vi "get_screen_resolution.vi"() -> (0 "Vertical Offset":i32, 1 "Height pixels":i16, 2 "Width pixels":i16)   [LabVIEW 2018]
uses:
  user32.dll
panel:
  out "Taskbar Height":i16
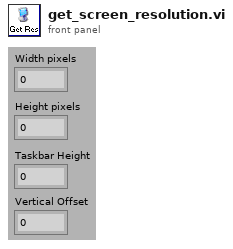
[diagram p1: front panel]
types:
  T1 = typedef "LVAllMonitorsDisplayTypeDef.ctl" = cluster{"Bounds":cluster{"Left":i16, "Top":i16, "Right":i16, "Bottom":i16}, "Depth":i16}[]
  T2 = typedef "LVRectTypeDef.ctl" = cluster{"Left":i16, "Top":i16, "Right":i16, "Bottom":i16}
  T3 = cluster{"Bounds":cluster{"Left":i16, "Top":i16, "Right":i16, "Bottom":i16}, "Depth":i16}
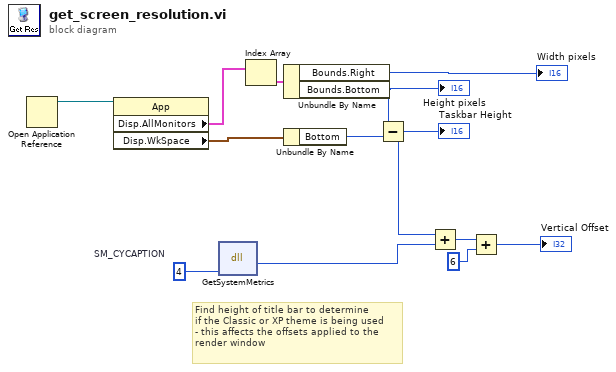
[diagram p0: block diagram]
diagram:
  w8 = 4  # SM_CYCAPTION
  # "Find height of title bar to determine\nif the Classic or XP theme is being used\n- this affects the offsets applied to the\nrender window"
  n1 = Open Application Reference() -> (3:w13:refnum<vi>)  [unwired: 1 in, 4 out]
  n2 = property class="App"(reference=w13) -> ("Disp.AllMonitors"=w12:T1, "Disp.WkSpace"=w10:T2)  [unwired: 1 in, 2 out]
  n3 = dll-call lib="user32.dll" fn="GetSystemMetrics" label="SetWindowPos"("parameter"=w8) -> ("return"=w4:i32)  [unwired: 4 in, 2 out]
  n4 = Index Array(array=w12) -> (element=w11:T3)  [unwired: 1 in]
  n5 = Unbundle By Name(w11) -> ("Bounds.Right"=→"Width pixels":i16, "Bounds.Bottom"=w6:i16)
  "Height pixels" <- w6
  n6 = Unbundle By Name(w10) -> ("Bottom"=w9:i16)
  n7 = Subtract(x=w6, y=w9) -> (x-y=w5:i16)
  "Taskbar Height" <- w5
  n8 = Add(x=w5, y=w4) -> (x+y=w2:i32)
  n9 = Add(x=w2, y=6) -> (x+y=→"Vertical Offset":i32)
